vi "getVideo.vi"(8 "error in (no error)":errorcluster, 10 "Video Id":string, 11 "ThirdPartyYoutubeLib in":refnum<class "ThirdPartyYoutubeLib.lvclass">) -> (0 "error out":errorcluster, 2 "Video":refnum<class "Video.lvclass">, 3 "ThirdPartyYoutubeLib out":refnum<class "ThirdPartyYoutubeLib.lvclass">)   [LabVIEW 2017, in "ThirdPartyYoutubeLib.lvclass"]
uses:
  ThirdPartyYoutubeLib.lvclass
  Video Class/Video.lvclass
  ThirdPartyYoutubeLib.lvclass/ThirdPartyYoutubeLib.ctl
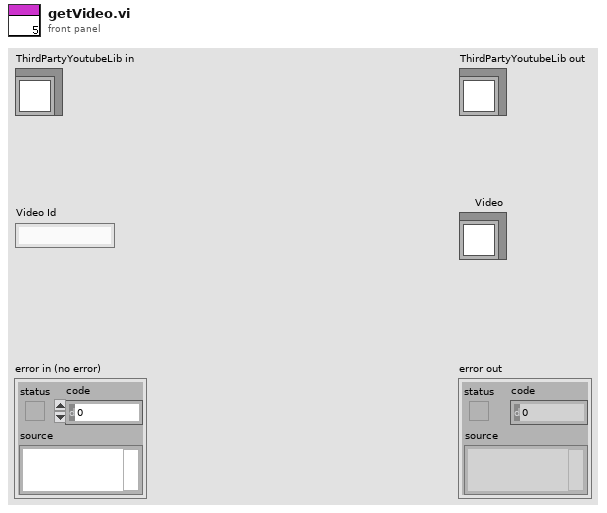
[diagram p1: front panel]
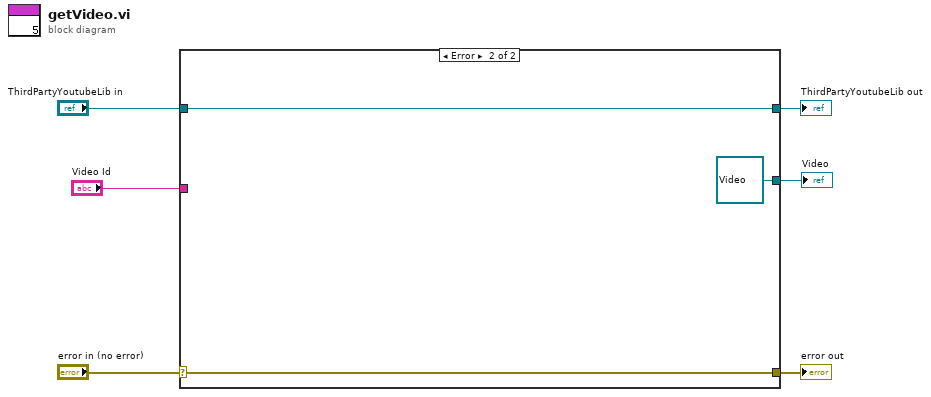
[diagram p0: block diagram]
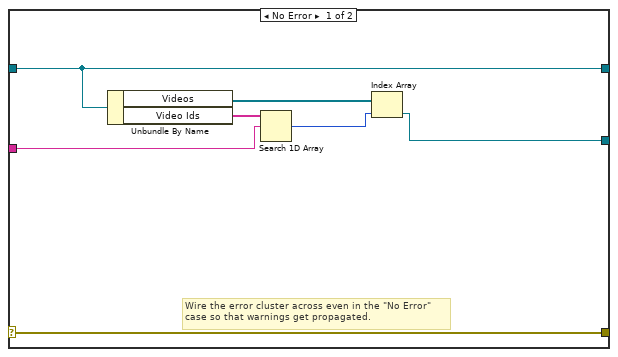
[diagram p2: hidden frame]
diagram:
  n1 = case shown="Error" "error in (no error)" {
    selector: "error in (no error)" -> [w13 w16]
    tunnel: [w13 w16] -> w5
    tunnel: [w12 w15] -> w3
    tunnel: "ThirdPartyYoutubeLib in" -> [w12 w15]
    tunnel: "Video Id" -> [w10 _]
    tunnel: [w7 refnum<class "Video.lvclass"> refnum ("Video")] -> w1
    frame No Error {
      # "Wire the error cluster across even in the \"No Error\"\ncase so that warnings get propagated."
      n2 = Unbundle By Name(w12) -> ("Videos"=w9:refnum<class "Video.lvclass">[], "Video Ids"=w11:string[])
      n3 = Search 1D Array(1D array=w11, element=w10) -> (index of element=w8:i32)  [unwired: 1 in]
      n4 = Index Array(array=w9, index=w8) -> (element=w7:refnum<class "Video.lvclass">)
    }
    frame Error {
    }
  }
  "error out" <- w5
  "ThirdPartyYoutubeLib out" <- w3
  "Video" <- w1
